vi "HMAC.vi"(5 "Output length (-1)":i32=-1, 7 "HASH-method":T1=enum."SHA-256" caption="HASH-method (SHA-256)", 8 "error in (no error)":errorcluster, 10 "Key":string, 11 "Message":string) -> (0 "error out":errorcluster, 1 "ASCII Formatted digest":string, 3 "HMAC digest (binary)":string)   [LabVIEW 2012, in "Encryption.lvlib"]
doc: "Calculates the HMAC bases on the <b>Message</b> and <b>Key</b>.\n\n(c) Ton Plomp, 2011\nTHIS SOFTWARE IS PROVIDED AS IS, AND ANY WARRANTY IS REJECTED"
uses:
  Encryption.lvlib
  hash-types.ctl
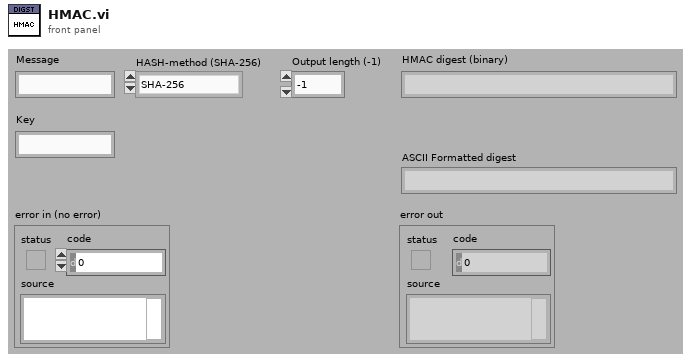
[diagram p1: front panel]
types:
  T1 = typedef "Encryption.lvlib/hash-types.ctl" = enum16{"MD5", "SHA-1", "SHA-224", "SHA-256", "SHA-384", "SHA-512"}
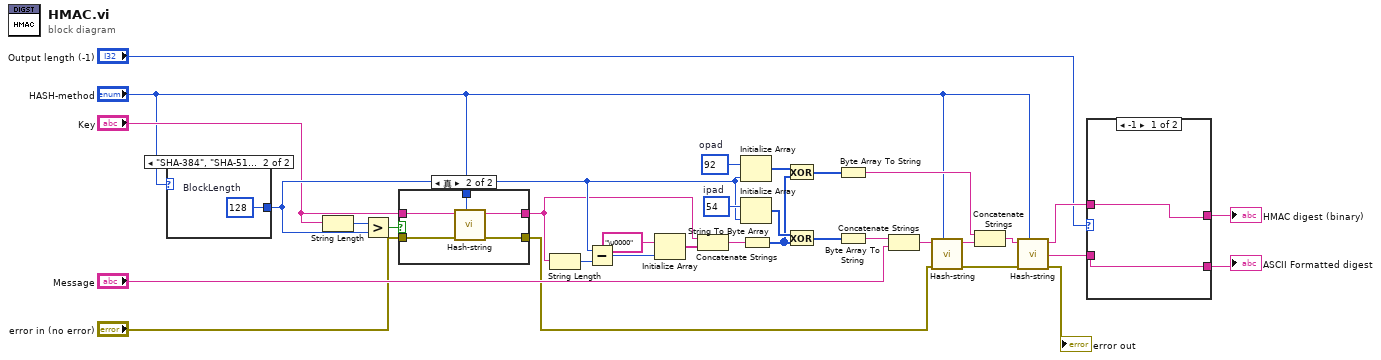
[diagram p0: block diagram]
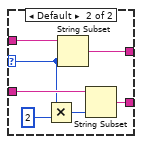
[diagram p2: hidden frame]
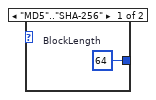
[diagram p4: hidden frame]
diagram:
  w26 = u8 92  # opad
  w33 = u8 54  # ipad
  n1 = case shown="\"SHA-384\", \"SHA-512\"" "HASH-method" {
    tunnel: [w34 w35] -> w12
    frame "MD5".."SHA-256" {
      w34 = 64  # BlockLength
    }
    frame "SHA-384", "SHA-512" {
      w35 = 128  # BlockLength
    }
  }
  n2 = String Length(string="Key") -> (length=w13:i32)
  n3 = Greater?(x=w13, y=w12) -> (0:w11:bool)
  n4 = case shown="真" w11 {
    tunnel: "Key" -> [w37 w41]
    tunnel: [w37 w38] -> w9
    tunnel: "HASH-method" -> [_ w42]
    tunnel: "error in (no error)" -> [w36 w40]
    tunnel: [w36 w39] -> w7
    frame False {
    }
    frame True {
      n5 = call "Hash-string.vi"("HASH-method"=w42, "error in (no error)"=w40, "Message"=w41) -> ("error out"=w39:errorcluster, "binary string hash"=w38:string)  [unwired: 6 in, 1 out]
    }
  }
  n6 = String Length(string=w9) -> (length=w32:i32)
  n7 = Subtract(x=w12, y=w32) -> (x-y=w30:i32)
  n8 = Initialize Array("\u0000", w30) -> (w29:string[])
  n9 = Concatenate Strings(w9, w29) -> (w28:string)
  n10 = Initialize Array(w26, w12) -> (w24:u8[])
  n11 = Initialize Array(w33, w12) -> (w27:u8[])
  n12 = String To Byte Array(string=w28) -> (unsigned byte array=w25:u8[])
  n13 = Exclusive Or(1:w25, 2:w24) -> (0:w18:u8[])
  n14 = Exclusive Or(1:w25, 2:w27) -> (0:w23:u8[])
  n15 = Byte Array To String(unsigned byte array=w18) -> (string=w19:string)
  n16 = Byte Array To String(unsigned byte array=w23) -> (string=w22:string)
  n17 = Concatenate Strings(w22, "Message") -> (w20:string)
  n18 = call "Hash-string.vi"("HASH-method"="HASH-method", "error in (no error)"=w7, "Message"=w20) -> ("error out"=w15:errorcluster, "binary string hash"=w17:string)  [unwired: 6 in, 1 out]
  n19 = Concatenate Strings(w19, w17) -> (w16:string)
  n20 = call "Hash-string.vi"("HASH-method"="HASH-method", "error in (no error)"=w15, "Message"=w16) -> ("error out"=→"error out":errorcluster, "ASCII formatted hash"=w4:string, "binary string hash"=w6:string)  [unwired: 6 in]
  n21 = case shown="-1" "Output length (-1)" {
    selector: "Output length (-1)" -> [_ w46]
    tunnel: w6 -> [w44 w51]
    tunnel: [w44 w50] -> w5
    tunnel: w4 -> [w43 w49]
    tunnel: [w43 w48] -> w3
    frame -1 {
    }
    frame Default {
      n22 = Multiply(x=w46, y=2) -> (x*y=w45:i32)
      n23 = String Subset(string=w51, length (rest)=w46) -> (substring=w50:string)  [unwired: 1 in]
      n24 = String Subset(string=w49, length (rest)=w45) -> (substring=w48:string)  [unwired: 1 in]
    }
  }
  "HMAC digest (binary)" <- w5
  "ASCII Formatted digest" <- w3
